vi "COMI WFM Rate Change.vi"(9 "nPPS":u32, 10 "ch":i32, 11 "hDevice":u32) -> (2 "function return":i32, 3 "hDevice out":u32)   [LabVIEW 2017, in "Comidll.lvlib"]
doc: "long (COMI_WFM_RateChange) (HANDLE hDevice, int ch, unsigned long nPPS);"
uses:
  <userlib>/Comidll/Comidll.lvlib
  <userlib>/Comidll/Comidll.dll
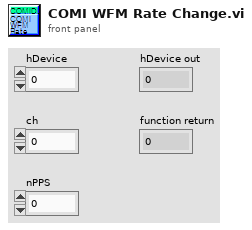
[diagram p1: front panel]
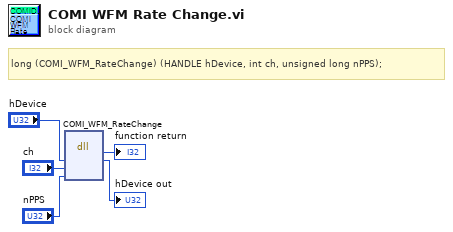
[diagram p0: block diagram]
diagram:
  # "long\t(COMI_WFM_RateChange) (HANDLE hDevice, int ch, unsigned long nPPS);"
  n1 = dll-call lib="C:/Program Files/National Instruments/LabVIEW 2017/user.lib/Comidll/Comidll.*" fn="COMI_WFM_RateChange"("hDevice"="hDevice", "ch"="ch", "nPPS"="nPPS") -> (→"function return":i32, "hDevice"=→"hDevice out":u32)  [unwired: 5 in, 2 out]
